vi "CarMove.vi"(7 "X done?":refnum<vi>, 8 "X+Y":i32=180, 9 "X":i32=80, 10 "speed":u32=1 min=1, 11 "Boolean in":refnum<vi>) -> ()   [LabVIEW 2024]
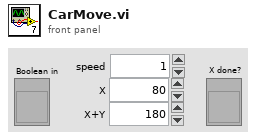
[diagram p1: front panel]
types:
  T1 = typedef "LVPositionTypeDef.ctl" = cluster{"Left":i32, "Top":i32}
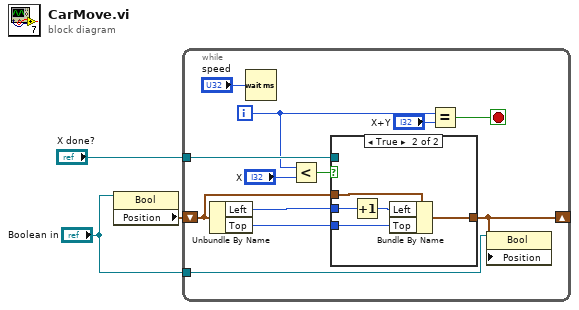
[diagram p0: block diagram]
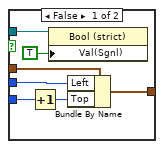
[diagram p2: hidden frame]
diagram:
  n1 = property on="Property Node" class="Bool"(reference="Boolean in") -> ("Position"=w3:T1)  [unwired: 1 in, 2 out]
  n2 = while {
    shift-right: [w12] -> _
    shift-left: w3 -> [w15]
    tunnel: "Boolean in" -> [w7]
    tunnel: "X done?" -> [w6]
    i -> [w4]
    stop <- w13 stop-if-true
    n3 = Unbundle By Name(w15) -> ("Left"=w11:i32, "Top"=w10:i32)
    n4 = Wait (ms)(milliseconds to wait="speed") -> ()  [unwired: 1 out]
    n5 = Less?(x=w4, y="X") -> (x < y?=w8:bool)
    n6 = case shown="True" w8 {
      tunnel: w15 -> [w19 w27]
      tunnel: [w20 w26] -> w12
      tunnel: w11 -> [w21 w25]
      tunnel: w10 -> [w22 w24]
      tunnel: w6 -> [w18 _]
      frame False {
        n7 = Increment(x=w22) -> (x+1=w16:i32)
        n8 = property on="Property Node" class="Bool (strict)"(reference=w18, "Val(Sgnl)"=TRUE ("Value")) -> ()  [unwired: 1 in, 2 out]
        n9 = Bundle By Name(cluster=w19, "Left"=w21, "Top"=w16) -> (w20:T1)
      }
      frame True {
        n10 = Increment(x=w25) -> (x+1=w23:i32)
        n11 = Bundle By Name(cluster=w27, "Left"=w23, "Top"=w24) -> (w26:T1)
      }
    }
    n12 = Equal?(x=w4, y="X+Y") -> (x = y?=w13:bool)
    n13 = property on="Property Node" class="Bool"(reference=w7, "Position"=w12) -> ()  [unwired: 1 in, 2 out]
  }
